vi "Notify.vi"(8 "Error In":errorcluster, 10 "Message":string, 11 "reference in":refnum<class "Customer.lvclass">) -> (0 "Error Out":errorcluster, 3 "reference in":refnum<class "Customer.lvclass">)   [LabVIEW 2020, in "Customer.lvclass"]
uses:
  Customer.lvclass
  Console_class/Console.lvclass
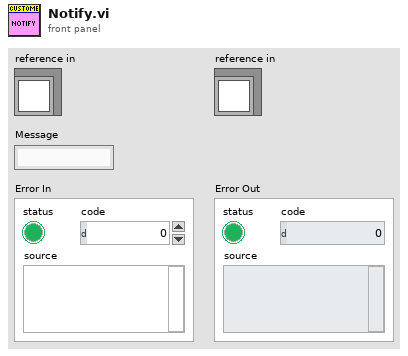
[diagram p1: front panel]
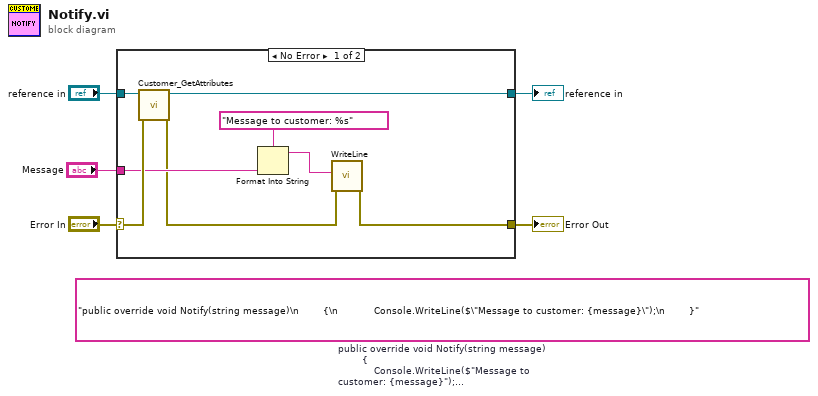
[diagram p0: block diagram]
diagram:
  (unwired) "public override void Notify(string message)\n        {\n            Console.WriteLine($\"Message to customer: {message}\");\n        }"  # public override void Notify(string message)         {             Console.WriteLine($"Message to customer: {message}");         }
  n1 = case shown="No Error" "Error In" {
    selector: "Error In" -> [w12 w15]
    tunnel: [w6 w15] -> w4
    tunnel: [w11 w14] -> w2
    tunnel: "reference in" -> [w13 w14]
    tunnel: "Message" -> [w9 _]
    frame No Error {
      n2 = call "Customer_GetAttributes.vi"("error in (no error)"=w12, "reference in"=w13) -> ("error out"=w7:errorcluster, "reference out"=w11:refnum<class "Customer.lvclass">)  [unwired: 6 in, 2 out]
      n3 = Format Into String(format string="Message to customer: %s", w9) -> (resulting string=w8:string)  [unwired: 2 in, 1 out]
      n4 = call "WriteLine.vi"("Error In"=w7, "ConsoleText"=w8) -> ("Error Out"=w6:errorcluster)  [unwired: 9 in]
    }
    frame Error {
    }
  }
  "Error Out" <- w4
  "reference in" <- w2
